vi "DataLogger.destructor.vi"(0 "i ref in":refnum<vi>, 5 "error in (no error)":errorcluster) -> (19 "error out":errorcluster)   [LabVIEW 2014, in "DataLogger.lvlib"]
doc: "This is the destructor of a class.\n\nLicense Agreement for this software:\n\nCopyright (C)\nGesellschaft für Schwerionenforschung, GSI\nPlanckstr. 1\n64291 Darmstadt\nGermany\n\nContact: D.Beck@gsi.de \n\nThis program is free software; you can redistribute it and/or modify it under the terms of the \nGNU General Public License as published by the Free Software Foundation; either version 2 of \nthe license, or (at your option) any later version.\n\nThis program is distributed in the hope that it will be useful, but WITHOUT ANY WARRANTY; \nwithout even the implied warranty of MERCHANTABILITY or FITNESS FOR A PARTICULAR PURPOSE. See the GNU General License for more details (http://www.gnu.org).\n\nGesellschaft für Schwerionenforschung, GSI\nPlanckstr. 1, 64291 Darmstadt, Germany\nFor all questions and ideas contact: M.Richter@gsi.de, H.Brand@gsi.de or D.Beck@gsi.de.\nLast update: 16-JUN-2004"
uses:
  DataLogger.lvlib
  CS_Core/CSApplicationBaseClasses/DeviceBase/DeviceBase.lvlib
  CSlibraries-extern/DimLVEvent/LVDimInterface/LVDimInterface.lvlib
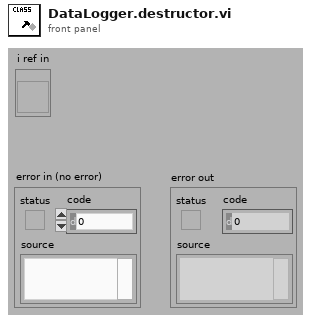
[diagram p1: front panel]
types:
  T1 = typedef "DataLogger.lvlib/DataLogger.i attribute.ctl" = cluster{"Service Names":string[], "Path":string[], "Service Alarm Index":i32[], "Service Alarm Limit1":dbl[], "Service Alarm Limit2":dbl[], "Service Alarm Indicator":bool[], "alarmID":i32, "pathID":i32, "SoundDeviceID":i32, "SoundFile":string, "SoundID":i32, "SoundFileID":i32}
  T2 = enum16{"SetAttribute", "GetAttribute", "CreateAttribute", "DestroyAttribute", "DestroyAllAtributes"}
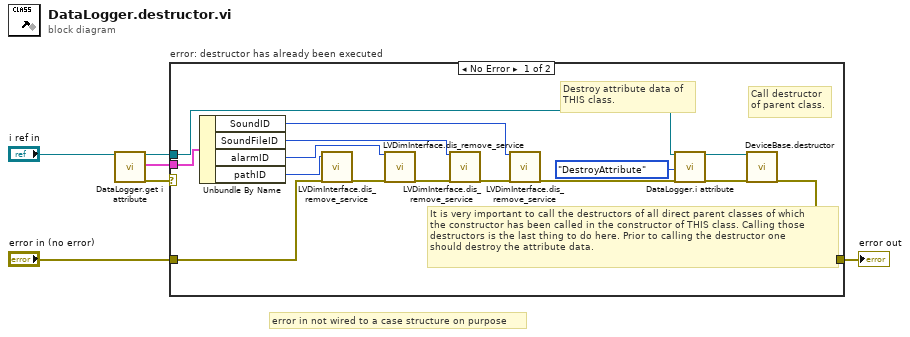
[diagram p0: block diagram]
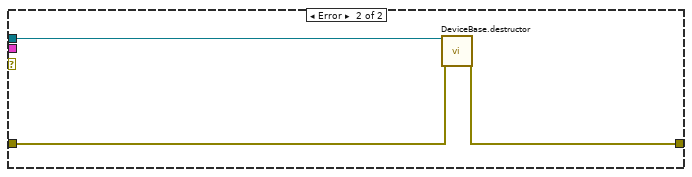
[diagram p2: hidden frame]
diagram:
  # "error in not wired to a case structure on purpose"
  n1 = call "DataLogger.get i attribute.vi"("i ref in"="i ref in") -> ("i ref out"=w2:refnum<vi>, "i attribute"=w1:T1, "error out"=w3:errorcluster)  [unwired: 16 in]
  n2 = case "error: destructor has already been executed" shown="No Error" w3 {
    tunnel: [w18 w22] -> w6
    tunnel: "error in (no error)" -> [w16 w23]
    tunnel: w2 -> [w12 w24]
    tunnel: w1 -> [w17 _]
    frame No Error {
      # "It is very important to call the destructors of all direct parent classes of which\nthe constructor has been called in the constructor of THIS class. Calling those\ndestructors is the last thing to do here. Prior to calling the destructor one \nshould destroy the attribute data."
      # "Destroy attribute data of \nTHIS class."
      # "Call destructor\nof parent class."
      n3 = Unbundle By Name(w17) -> ("SoundID"=w7:i32, "SoundFileID"=w8:i32, "alarmID"=w14:i32, "pathID"=w13:i32)
      n4 = call "LVDimInterface.dis_remove_service.vi"("my_serviceID"=w13, "error in (no error)"=w16) -> ("error out"=w15:errorcluster)  [unwired: 17 in]
      n5 = call "LVDimInterface.dis_remove_service.vi"("my_serviceID"=w14, "error in (no error)"=w15) -> ("error out"=w11:errorcluster)  [unwired: 17 in]
      n6 = call "LVDimInterface.dis_remove_service.vi"("my_serviceID"=w8, "error in (no error)"=w11) -> ("error out"=w10:errorcluster)  [unwired: 17 in]
      n7 = call "LVDimInterface.dis_remove_service.vi"("my_serviceID"=w7, "error in (no error)"=w10) -> ("error out"=w9:errorcluster)  [unwired: 17 in]
      n8 = call "DataLogger.i attribute.vi"("VI Refnum"=w12, "Action"=T2."DestroyAttribute", "error in (no error)"=w9) -> ("VI Refnum out"=w20:refnum<vi>, "error out"=w19:errorcluster)  [unwired: 14 in, 1 out]
      n9 = call "DeviceBase.destructor.vi"("i ref in"=w20, "error in (no error)"=w19) -> ("error out"=w18:errorcluster)  [unwired: 17 in]
    }
    frame Error {
      n10 = call "DeviceBase.destructor.vi"("i ref in"=w24, "error in (no error)"=w23) -> ("error out"=w22:errorcluster)  [unwired: 17 in]
    }
  }
  "error out" <- w6
